vi "AudioTest.Manager.vi"(11 "Module Config":T4={"Name"="Audio Test", "Parent Q"=refnum, "Is Child?"=FALSE, "Index"=0, "Dirs"={"Root"=path "", "Config"=path "C:/ATE/Config", "Logs"=path "C:/ATE/Logs", "Reports"=path "C:/ATE/Reports", "App Data"=path "C:/ProgramData/MAIN"}, "Simulate"=FALSE, "SimCtrl"=refnum}) -> ()   [LabVIEW 2018]
uses:
  <vilib>/KATE/Module/Module Config.ctl
  <vilib>/KATE/Queues/Q.Element.ctl
  <vilib>/KATE/Module/Module.Working Dirs.ctl
  <vilib>/KATE/Event Log/Event Notification/Event Log.Log Level.ctl
  <vilib>/sound2/lvsound2.llb/Sound Data Format.ctl
  <vilib>/KATE/Module/Module.SW Version Info.ctl
  <vilib>/KATE/Module/Window/Window.Task, Action.ctl
  Utils/Functions/FunctMgr/FunctMgr.lvclass
  <vilib>/sound2/lvsound2.llb/Sound Input Task ID.ctl
  <vilib>/sound2/lvsound2.llb/Sampling Mode.ctl
  <vilib>/Utility/sysdir.llb/System Directory Type.ctl
  <vilib>/KATE/Event Log/Event Notification/Event Log.Notification Type.ctl
  <vilib>/sound2/lvsound2.llb/Sound Input Read (DBL).vi
  <vilib>/measure/maspectr.llb/FFT Spectrum (Mag-Phase) for 1 Chan.vi
  <vilib>/KATE/Config/Stored Controls/Class.SaveCtrls.lvclass
  <vilib>/KATE/Queues/Queue Utils.lvlib
  <vilib>/KATE/Module/Module Utils.lvlib
  <vilib>/KATE/Event Log/Event Log.lvlib
  <vilib>/KATE/Scheduler/Scheduler.lvlib
  <vilib>/KATE/Menu/Menu Utils.lvlib
  <vilib>/KATE/Config/Config Utils.lvlib
  <vilib>/KATE/Status/Status Utils.lvlib
  <vilib>/KATE/Files/File Utils.lvlib
  <vilib>/KATE/SeqMgr/SeqMgr.lvlib
  <vilib>/KATE/Event Log/Event Notification/Event Notification.lvclass
  <vilib>/measure/NI_MAPro.lvlib
  <vilib>/KATE/Time/Time Utils.lvlib
panel:
  in  "Main Tab":enum32{"Operate", "Maint"}(tab)
  in  "Data Tab":enum32{"Control", "Config"}(tab)
  out "Dur(s)":dbl=1.0 min=0.1 max=10.0
  out "Recording":bool
  in  "Interval(s)":dbl=1.0 min=0.1 max=10.0
  in  "Read Audio":bool
  in  "Read Baseline":bool
  in  "Save Data to File":bool
  out "Status":string
  in  "Limits":T1(array[cluster])=[{"FreqStart"=0.0, "FreqEnd"=1000.0, "Lim_dB"=-45.0, "Result"=TRUE}, {"FreqStart"=1000.0, "FreqEnd"=8000.0, "Lim_dB"=-60.0, "Result"=TRUE}] {"Lim_dB" format="%#_6f"; "FreqEnd" format="%#.3f"; "FreqStart" format="%#.3f"}
  out "FFT":cluster{"f0":dbl, "df":dbl, "magnitude":dbl[]}[](graph)
  in  "Toggle Sim":bool
  out "Error":errorcluster
  in  "Logging Level":T2
  in  "Audio Format":T3={"sample rate (S/s)"=22050.0, "number of channels"=2, "bits per sample"=16}
  out "Rev":string="v1.0.0"
  out "Simulate Indication":string="Simulating Instruments"
  out "Error Status":string
  in  "Clear Error":bool
  in  "Leave Maint":bool
  # "Audio Test"
  # "Start(Hz)         End(Hz)                    Limit"
  # "P/F"
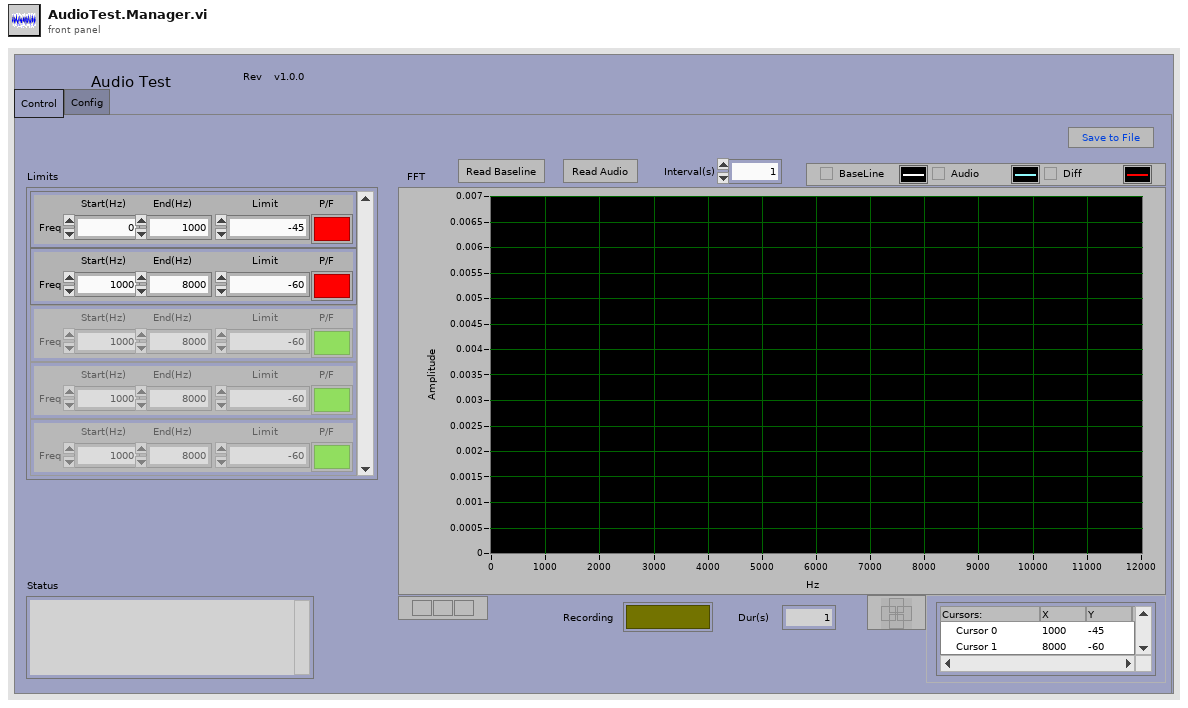
[diagram p1: front panel]
types:
  T1 = cluster{"FreqStart":dbl, "FreqEnd":dbl, "Lim_dB":dbl, "Result":bool}[]
  T2 = typedef "KATE_Lib.lvlib/Event Log.lvlib/Event Log.Log Level.ctl" = enum16{"Normal", "Verbose", "Debug0", "Debug1", "Debug2"}
  T3 = typedef "Sound Data Format.ctl" = cluster{"sample rate (S/s)":dbl, "number of channels":i32, "bits per sample":i32}
  T4 = typedef "KATE_Lib.lvlib/Module Utils.lvlib/Module Config.ctl" = cluster{"Name":string, "Parent Q":refnum<queue>, "Is Child?":bool, "Index":i32, "Dirs":T5, "Simulate":bool, "SimCtrl":refnum<vi>}
  T5 = typedef "KATE_Lib.lvlib/Module Utils.lvlib/Module.Working Dirs.ctl" = cluster{"Root":path, "Config":path, "Logs":path, "Reports":path, "App Data":path}
  T6 = typedef "KATE_Lib.lvlib/Module Utils.lvlib/Module.SW Version Info.ctl" = cluster{"AppName":string, "Company":string, "Version":string, "Description":string, "PN":string}
  T7 = typedef "KATE_Lib.lvlib/Module Utils.lvlib/Module Sys Info.ctl" = cluster{"Main Q":refnum<queue>, "Exe":bool, "SW Rev":T6, "Self Ref":refnum<vi>, "Main Tab":refnum<vi>, "Pane":refnum<vi>, "Stop":cluster{"Ref":refnum<event-registration>, "Event":refnum<user-event>}, "Cfg":T4, "Services":cluster{"Name":string, "vi ref":refnum<vi>}[], "Menu Ref":refnum<k9>, "CtrlStates":refnum<class "Class.SaveCtrls.lvclass">, "Docs":cluster{"Tags":string[], "Paths":path[]}, "Log":refnum<class "Event Notification.lvclass">, "Test Controls":refnum<vi>[], "Child Modules":cluster{"Name":string, "vi ref":refnum<vi>}[], "SW Items":string[][], "AppData":refnum<class "Class.AppData.lvclass">}
  T8 = enum8{"Enabled", "Disabled", "Disabled and Grayed Out"}
  T9 = cluster{"dB On (F)":bool, "unwrap phase (F)":bool, "convert to degree (F)":bool}
  T10 = enum16{"open", "replace", "create", "open or create", "replace or create", "replace or create with confirmation"}
  T11 = cluster{"FreqStart":dbl, "FreqEnd":dbl, "Lim":dbl, "Result":bool}
  T12 = typedef "KATE_Lib.lvlib/Event Log.lvlib/Event Log.Notification Type.ctl" = enum16{"Normal", "Warning", "Error", "Success"}
  T13 = typedef "Sound Input Task ID.ctl" = u32
  T14 = cluster{"Child Modules":cluster{"VI Ref":refnum<vi>, "Name":string}[]}
  T15 = cluster{"Local Error":errorcluster, "Lnch":bool, "FunctMgr":refnum<class "FunctMgr.lvclass">, "App":cluster{"Child Modules":cluster{"VI Ref":refnum<vi>, "Name":string}[]}, "Task ID":T13, "GraphData":cluster{"t":dbl[], "Y":dbl[]}, "Baseline":cluster{"f0":dbl, "df":dbl, "magnitude":dbl[]}, "Audio":cluster{"f0":dbl, "df":dbl, "magnitude":dbl[]}, "Diff":cluster{"f0":dbl, "df":dbl, "magnitude":dbl[]}}
  T16 = typedef "Sampling Mode.ctl" = i32
  T17 = cluster{"FreqStart":dbl, "FreqEnd":dbl, "Lim_dB":dbl, "Result":bool}
  T18 = typedef "System Directory Type.ctl" = i32
  T19 = typedef "KATE_Lib.lvlib/Module Utils.lvlib/Window.Task, Action.ctl" = enum16{"Resize()", "Show Panel(Bool)", "Show Scroll Bars(Bool)", "Dock to SubPanel(SubPanel Ref)", "Undock from SubPanel()", "Return to SubPanel()", "Go To Maint Tab()", "Show Maint Tab(Bool)", "Open Block Diagram()"}
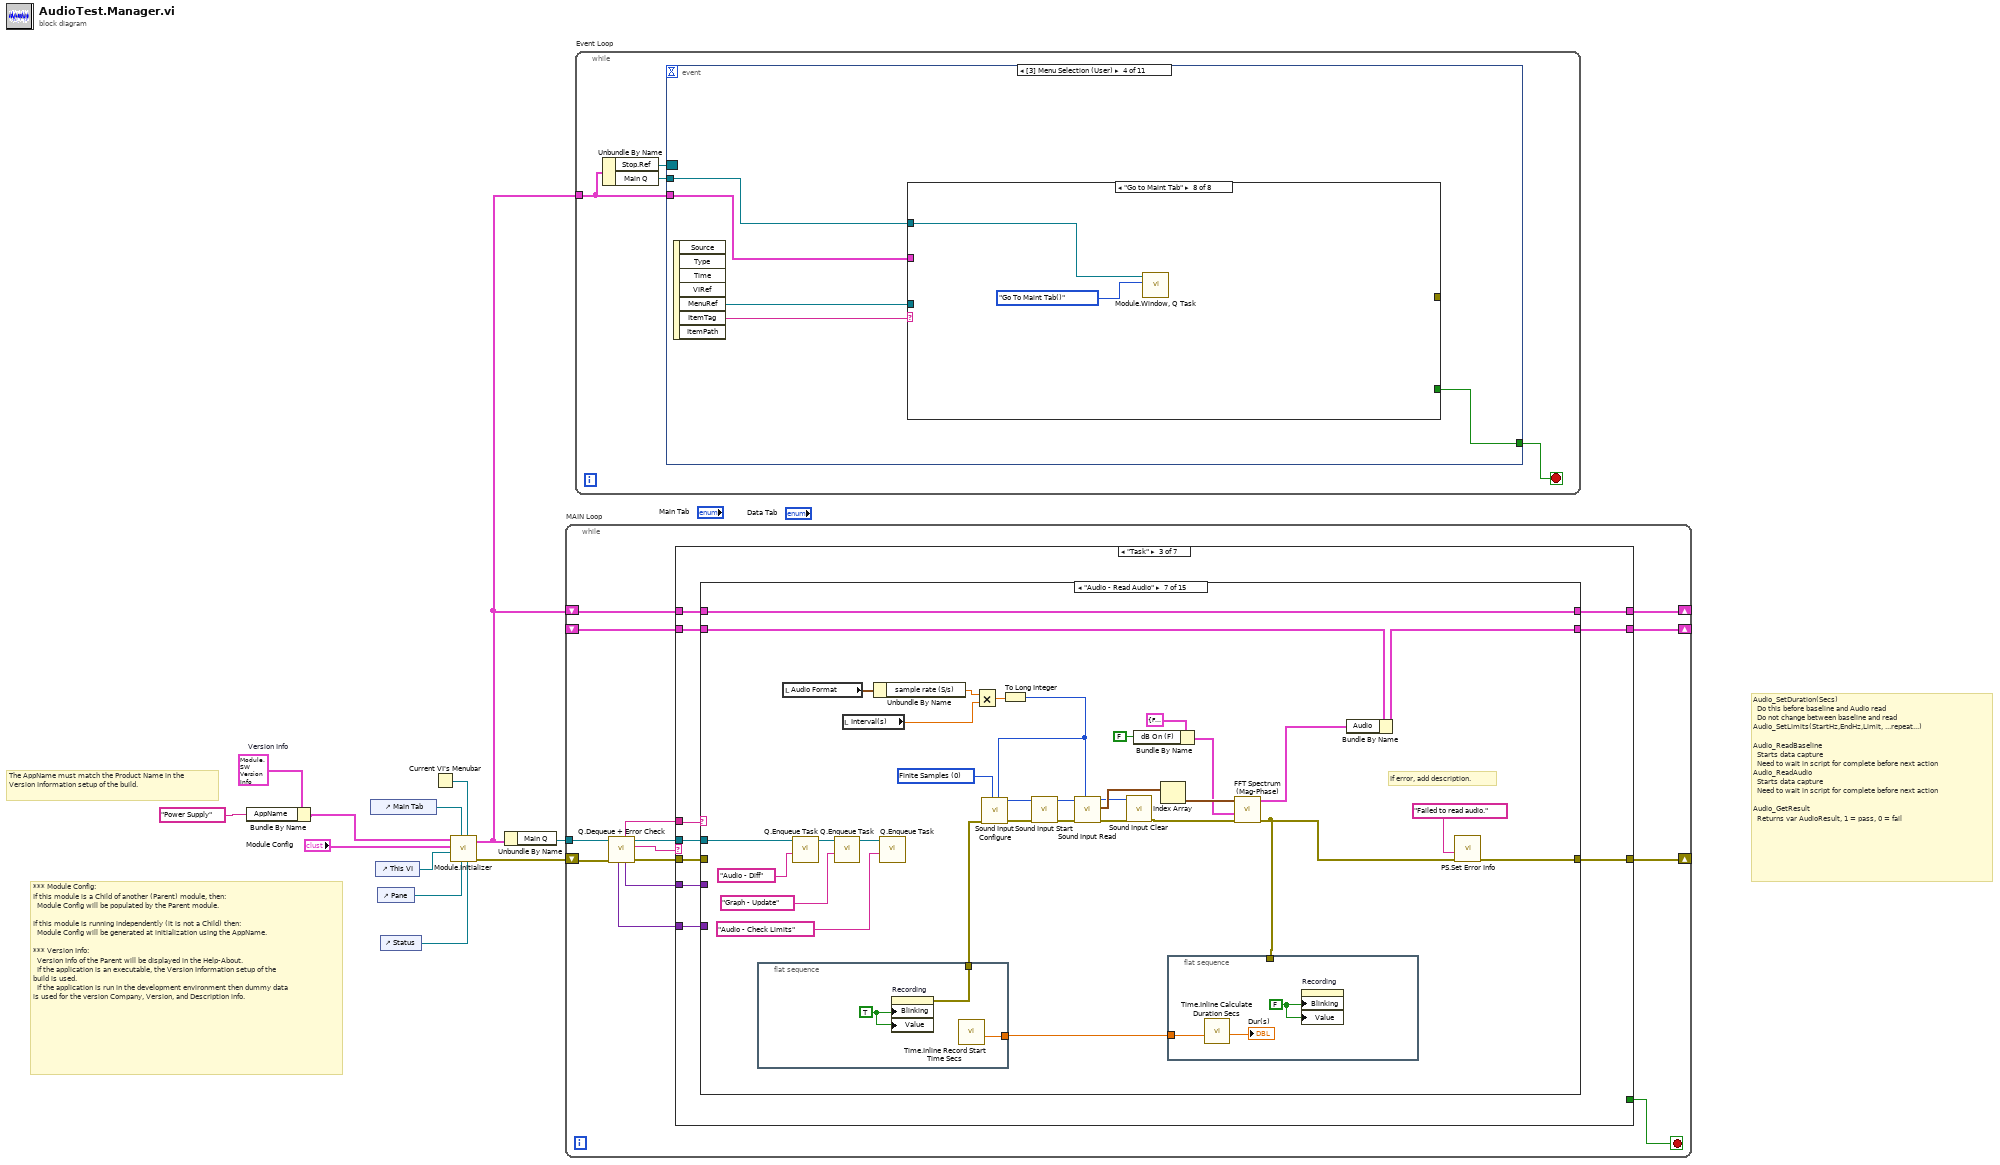
[diagram p0: block diagram]
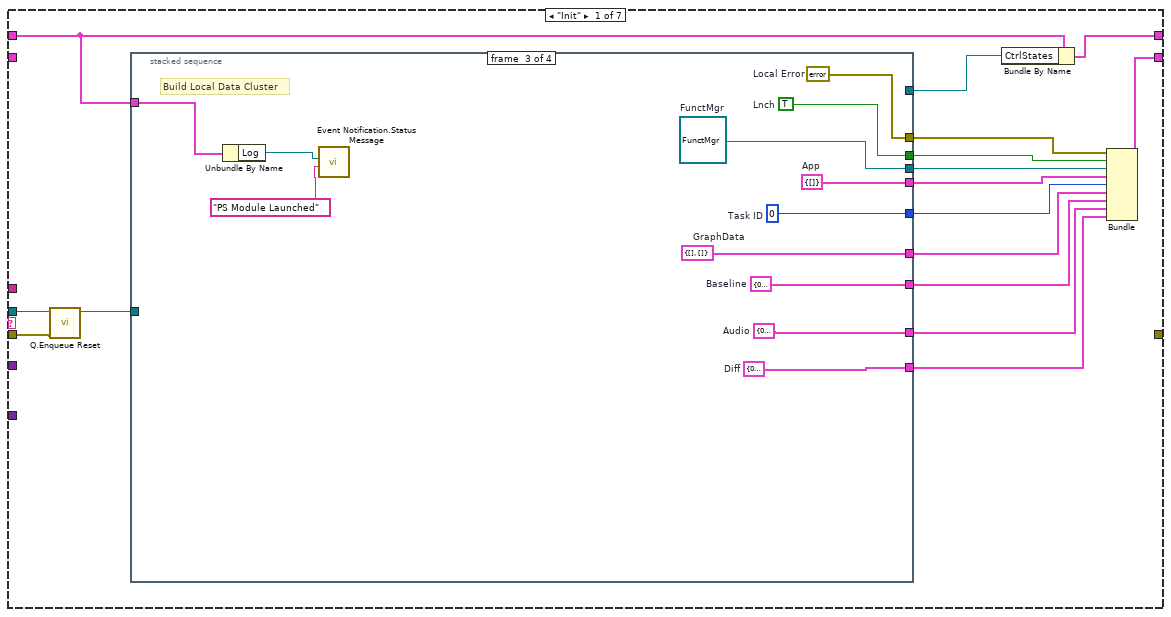
[diagram p2: hidden frame]
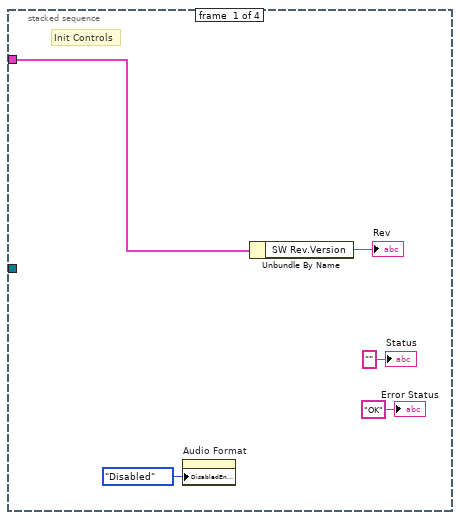
[diagram p3: hidden frame]
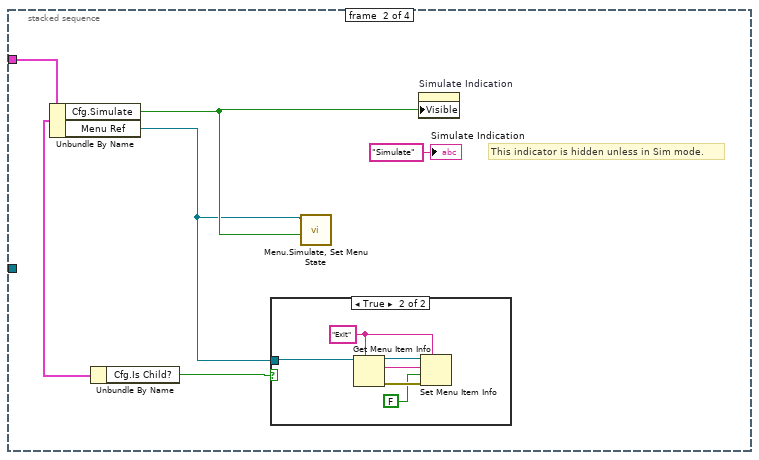
[diagram p4: hidden frame]
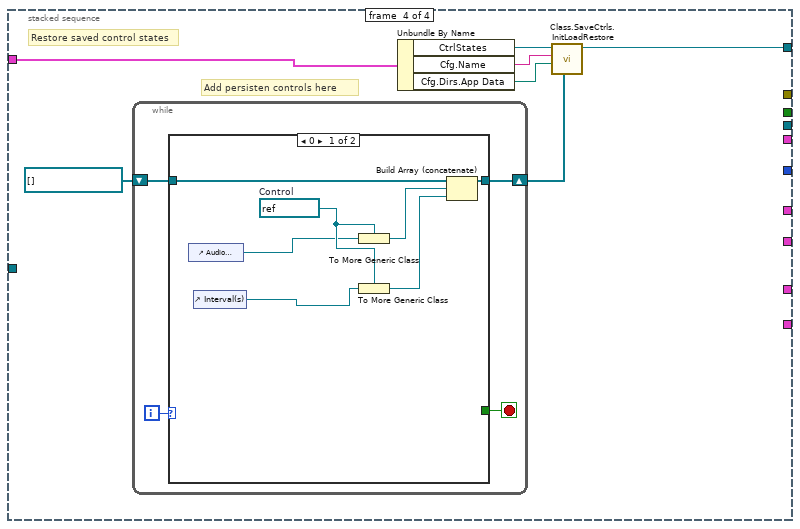
[diagram p6: hidden frame]
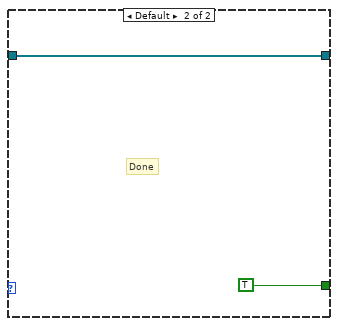
[diagram p7: hidden frame]
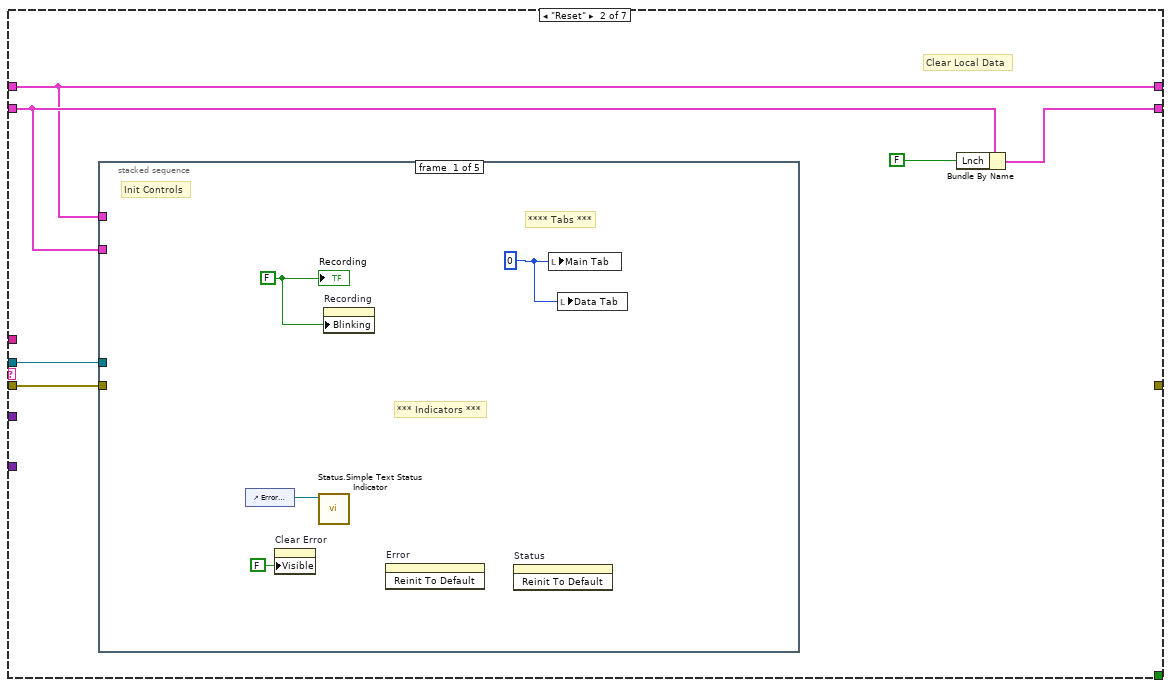
[diagram p8: hidden frame]
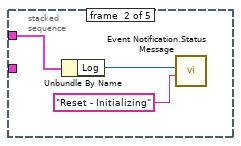
[diagram p9: hidden frame]
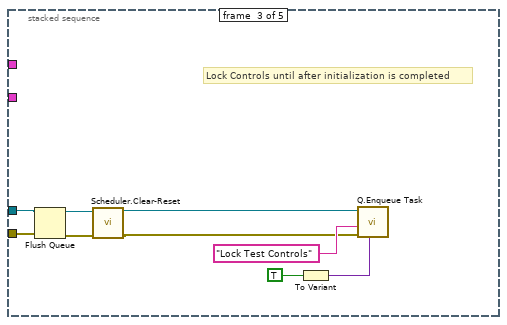
[diagram p10: hidden frame]
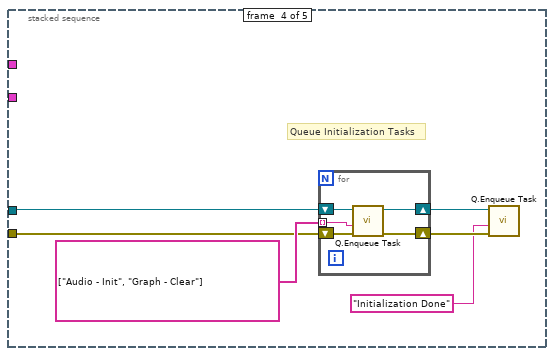
[diagram p11: hidden frame]
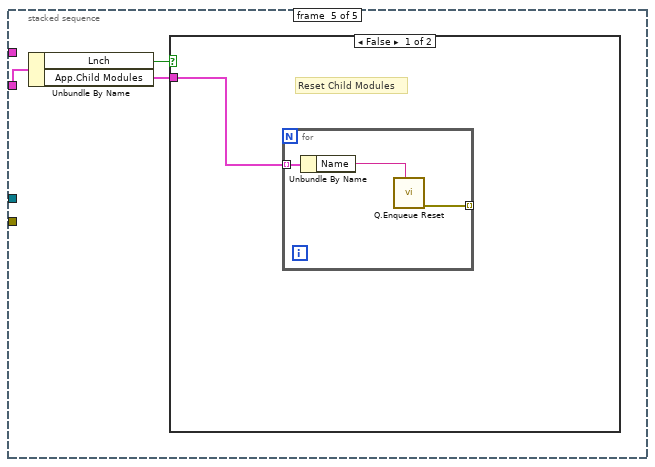
[diagram p12: hidden frame]
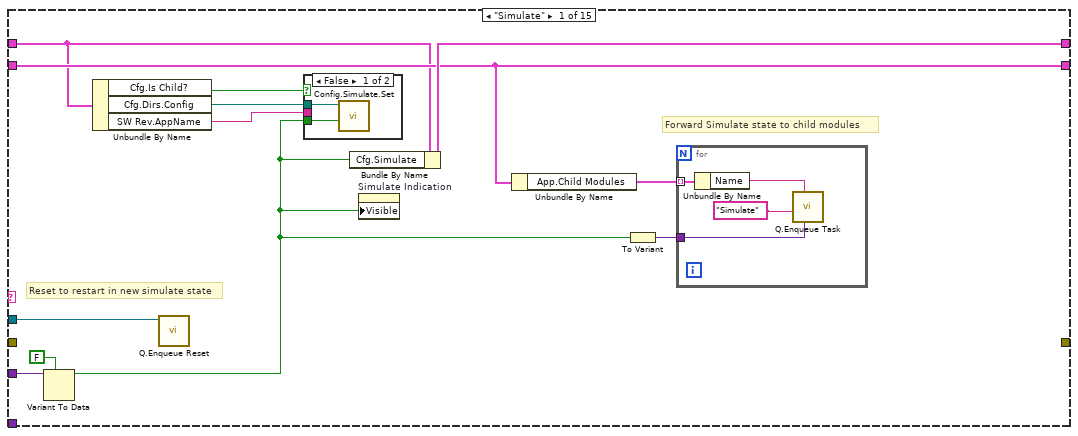
[diagram p14: hidden frame]
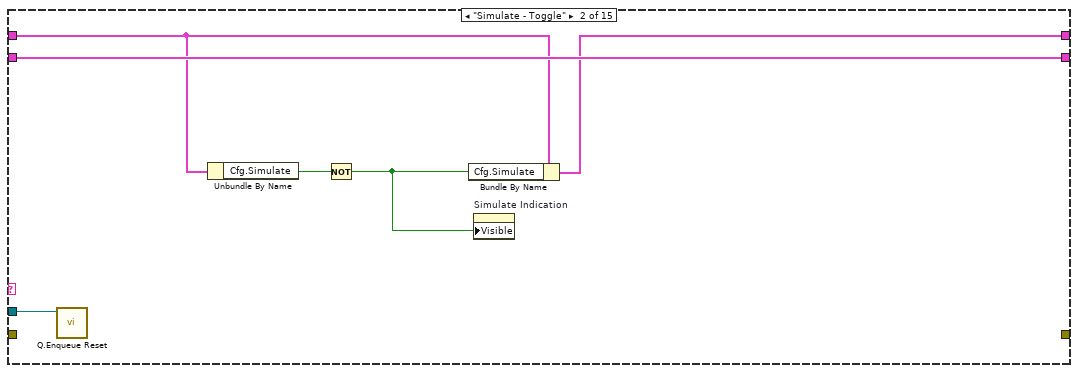
[diagram p16: hidden frame]
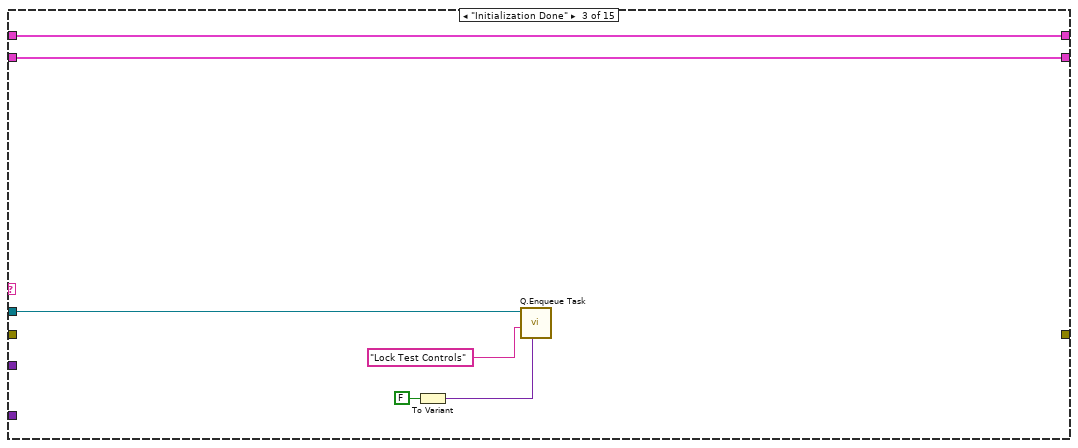
[diagram p17: hidden frame]
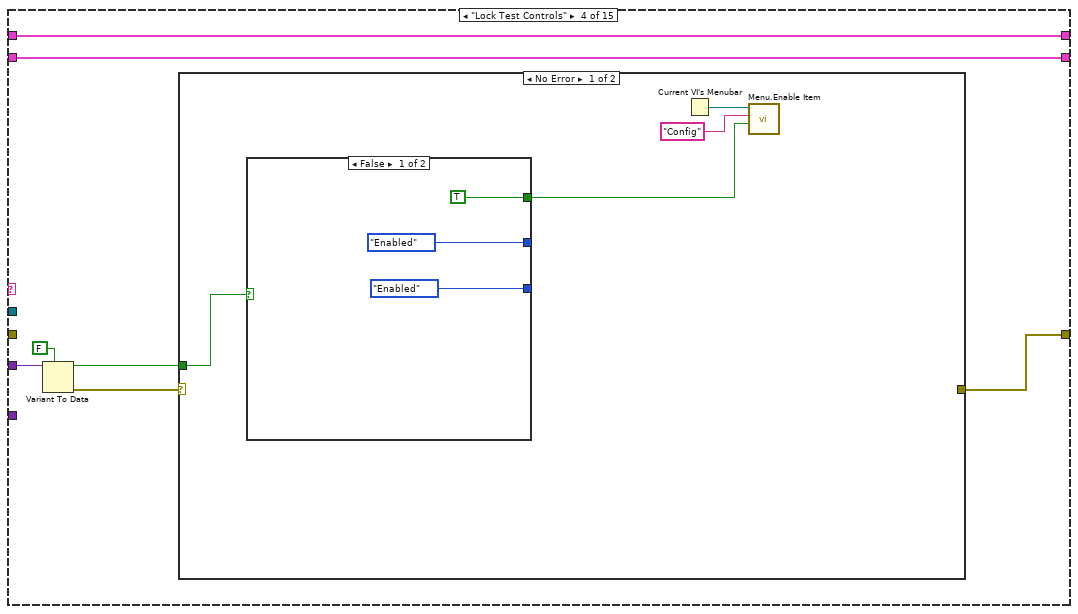
[diagram p18: hidden frame]
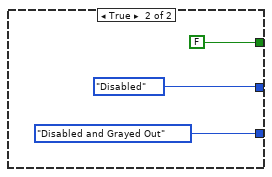
[diagram p19: hidden frame]
diagram:
  w2 = T6 {"AppName"="ModuleX", "Company"="CompanyX", "Version"="1.0", "Description"="This app is being developed.", "PN"=""}  # Version Info
  # "Audio_SetDuration(Secs)\n  Do this before baseline and Audio read\n  Do not change between baseline and read\nAudio_SetLimits(StartHz,EndHz,Limit, ...repeat...)\n\nAudio_ReadBaseline\n  Starts data capture\n  Need to wait in script for complete before next action\nAudio_ReadAudio\n  Starts data capture\n  Need to wait in script for complete before next action\n\nAudio_GetResult\n  Returns var AudioResult, 1 = pass, 0 = fail"
  # "*** Module Config:\nIf this module is a Child of another (Parent) module, then:\n  Module Config will be populated by the Parent module.\n\nIf this module is running independently (it is not a Child) then:\n  Module Config will be generated at initialization using the AppName.\n\n*** Version Info:\n  Version Info of the Parent will be displayed in the Help-About.\n  If the application is an executable, the Version Information setup of the build is used.\n  If the application is run in the development environment then dummy data is used for the version Company, Version, and Description info."
  # "The AppName must match the Product Name in the Version Information setup of the build."
  n1 = Bundle By Name(cluster=w2, "AppName"="Power Supply") -> (w1:T6)
  n2 = control-ref of="Main Tab"() -> (w10:refnum<vi>)
  n3 = control-ref of="This VI"() -> (w9:refnum<vi>)
  n4 = control-ref of="Pane"() -> (w8:refnum<vi>)
  n5 = control-ref of="Status"() -> (w4:refnum<vi>)
  n6 = Current VI's Menubar() -> (w6:refnum<k9>)
  n7 = call <vilib>:"Module.Initializer.vi"("StatusTxtBx"=w4, "Menu Ref"=w6, "Pane"=w8, "Main Tab"=w10, "Self Ref"=w9, "Module Config"="Module Config", "SW Rev"=w1) -> ("error out"=w12:errorcluster, "Sys"=w7:T7)  [unwired: 3 in]
  n8 = Unbundle By Name(w7) -> ("Main Q"=w11:refnum<queue>)
  n9 = while "MAIN Loop" {
    shift-right: [w23] -> _
    shift-left: w12 -> [w21]
    shift-right: [w24] -> _
    shift-left: _ -> [w13]
    shift-right: [w25] -> _
    shift-left: w7 -> [w26]
    tunnel: w11 -> [w20]
    stop <- w15 stop-if-true
    n10 = call <vilib>:"Q.Dequeue + Error Check.vi"("Error In"=w21, "Q In"=w20) -> ("error out"=w22:errorcluster, "Cmd"=w19:string, "Q Out"=w18:refnum<queue>, "Data1"=w17:variant, "Sub"=w14:string, "Data2"=w16:variant)  [unwired: 4 in]
    n11 = case shown="\"Task\"" w19 {
      selector: w19 -> [_ _ _ _ _ w508 _]
      tunnel: w13 -> [_ w93 w139 w407 w482 w502 w567]
      tunnel: w26 -> [w37 w91 w140 w408 w483 w503 w568]
      tunnel: [w38 w91 w138 w406 w481 w503 w568] -> w25
      tunnel: [w40 w96 w137 w405 w480 w501 w567] -> w24
      tunnel: [_ _ w131 w400 _ w509 w570] -> w23
      tunnel: w22 -> [w41 w94 w133 w401 _ w506 _]
      tunnel: w18 -> [w42 w95 w134 w402 w486 w504 _]
      tunnel: w17 -> [_ _ w135 w403 w485 w507 _]
      tunnel: w16 -> [_ _ w132 w399 w484 _ _]
      tunnel: w14 -> [_ _ w136 w404 w487 w505 _]
      tunnel: [_ _ _ _ _ _ TRUE] -> w15
      frame "Init" {
        n12 = call <vilib>:"Q.Enqueue Reset.vi"("Error In"=w41, "Q In"=w42) -> ("Q Out"=w35:refnum<queue>)  [unwired: 8 in, 1 out]
        n13 = stacked-sequence {
          tunnel: [_ _ w64 _] -> w39
          tunnel: w37 -> [w46 w49 w67 w72]
          tunnel: [_ _ _ w71] -> w36
          tunnel: w35 -> [_ _ _ _]
          tunnel: [_ _ w70 _] -> w34
          tunnel: [_ _ w69 _] -> w33
          tunnel: [_ _ w62 _] -> w32
          tunnel: [_ _ w68 _] -> w31
          tunnel: [_ _ w63 _] -> w30
          tunnel: [_ _ w61 _] -> w29
          tunnel: [_ _ w60 _] -> w28
          tunnel: [_ _ w59 _] -> w27
          frame #0 {
            # "Init Controls"
            n14 = property on="Audio Format" class="Clust (strict)"("DisabledEnum"=T8."Disabled" ("Disabled")) -> ()  [unwired: 2 in, 2 out]
            n15 = Unbundle By Name(w46) -> ("SW Rev.Version"=→"Rev":string)
            "Status" <- "" ("Status")
            "Error Status" <- "OK" ("Error Status")
          }
          frame #1 {
            # "This indicator is hidden unless in Sim mode."
            n16 = Unbundle By Name(w49) -> ("Cfg.Simulate"=w51:bool, "Menu Ref"=w48:refnum<k9>)
            n17 = Unbundle By Name(w49) -> ("Cfg.Is Child?"=w50:bool)
            n18 = case shown="True" w50 {
              tunnel: w48 -> [_ w54]
              frame False {
              }
              frame True {
                w56 = "Exit"
                n19 = Get Menu Item Info(7:w56, 11:w54) -> (0:w55:errorcluster, 2:w57:string, 3:w58:refnum<k9>)  [unwired: 1 in, 4 out]
                n20 = Set Menu Item Info(7:w56, 8:w55, 9:FALSE ("enabled"), 10:w57, 11:w58) -> ()  [unwired: 2 in, 2 out]
              }
            }
            n21 = call <vilib>:"Menu.Simulate, Set Menu State.vi"("Sim Enable"=w51, "Menu Ref"=w48) -> ()  [unwired: 8 in, 2 out]
            n22 = property on="Simulate Indication" class="Str"("Visible"=w51) -> ()  [unwired: 2 in, 2 out]
            "Simulate Indication" <- "Simulate" ("Simulate Indication")
          }
          frame #2 {
            w59 = cluster{"f0":dbl, "df":dbl, "magnitude":dbl[]} {"f0"=0.0, "df"=0.0, "magnitude"=[]}  # Diff
            w60 = cluster{"f0":dbl, "df":dbl, "magnitude":dbl[]} {"f0"=0.0, "df"=0.0, "magnitude"=[]}  # Audio
            w61 = cluster{"f0":dbl, "df":dbl, "magnitude":dbl[]} {"f0"=0.0, "df"=0.0, "magnitude"=[]}  # Baseline
            w62 = T13 0  # Task ID
            w63 = cluster{"t":dbl[], "Y":dbl[]} {"t"=[], "Y"=[]}  # GraphData
            w68 = errorcluster {"status"=FALSE, "code"=0, "source"=""}  # Local Error
            w64 = refnum<class "FunctMgr.lvclass"> refnum  # FunctMgr
            w69 = T14 {"Child Modules"=[]}  # App
            w70 = TRUE  # Lnch
            # "Build Local Data Cluster"
            n23 = Unbundle By Name(w67) -> ("Log"=w66:refnum<class "Event Notification.lvclass">)
            n24 = call <vilib>:"Event Notification.Status Message.vi"("Message"="PS Module Launched", "Event Notification in"=w66) -> ()  [unwired: 10 in]
          }
          frame #3 {
            # "Add persisten controls here"
            # "Restore saved control states"
            n25 = while {
              shift-right: [w79] -> w73
              shift-left: refnum<vi>[] [] -> [w80]
              i -> [w81]
              stop <- w78 stop-if-true
              n26 = case shown="0" w81 {
                tunnel: w80 -> [w87 w90]
                tunnel: [w88 w90] -> w79
                tunnel: [_ TRUE] -> w78
                frame 0 {
                  w84 = refnum<vi> refnum  # Control
                  n27 = control-ref of="Audio Format"() -> (w83:refnum<vi>)
                  n28 = control-ref of="Interval(s)"() -> (w82:refnum<vi>)
                  n29 = To More Generic Class(target class=w84, reference=w83) -> (generic class reference=w86:refnum<vi>)
                  n30 = To More Generic Class(target class=w84, reference=w82) -> (generic class reference=w85:refnum<vi>)
                  n31 = Build Array (concatenate)(w87, w86, w85) -> (w88:refnum<vi>[])
                }
                frame Default {
                  # "Done"
                }
              }
            }
            n32 = Unbundle By Name(w72) -> ("CtrlStates"=w74:refnum<class "Class.SaveCtrls.lvclass">, "Cfg.Name"=w76:string, "Cfg.Dirs.App Data"=w75:path)
            n33 = call-dynamic "Class.SaveCtrls.InitLoadRestore.vi"("Ctrl Array"=w73, "Module Data Dir"=w75, "Module Name"=w76, "CtrlStates In"=w74) -> ("CtrlStates"=w71:refnum<class "Class.SaveCtrls.lvclass">)  [unwired: 6 in, 1 out]
          }
        }
        n34 = Bundle By Name(cluster=w37, "CtrlStates"=w36) -> (w38:T7)
        n35 = Bundle("Local Error"=w31, "Lnch"=w34, "FunctMgr"=w39, "App"=w33, "Task ID"=w32, "GraphData"=w30, "Baseline"=w29, "Audio"=w28, "Diff"=w27) -> (w40:T15)  [unwired: 1 in]
      }
      frame "Reset" {
        # "Clear Local Data"
        n36 = stacked-sequence {
          tunnel: w95 -> [_ _ w105 w113 _]
          tunnel: w94 -> [_ _ w104 w117 _]
          tunnel: w93 -> [_ _ _ _ w126]
          tunnel: w91 -> [_ w103 _ _ _]
          frame #0 {
            w97 = FALSE ("Recording")
            w100 = 0
            # "*** Indicators ***"
            # "**** Tabs ***"
            # "Init Controls"
            n37 = control-ref of="Error Status"() -> (w99:refnum<vi>)
            n38 = property on="Clear Error" class="Bool"("Visible"=FALSE) -> ()  [unwired: 2 in, 2 out]
            n39 = call <vilib>:"Status.Simple Text Status Indicator.vi"("Status TextBox"=w99) -> ()  [unwired: 10 in, 1 out]
            n40 = property on="Recording" class="Bool (strict)"("Blinking"=w97) -> ()  [unwired: 2 in, 2 out]
            n41 = invoke on="Error" class="Clust (strict)" method="Reinit To Default"() -> ()  [unwired: 3 in, 3 out]
            n42 = invoke on="Status" class="Str" method="Reinit To Default"() -> ()  [unwired: 3 in, 3 out]
            n43 = local write "Main Tab"(w100) -> ()
            n44 = local write "Data Tab"(w100) -> ()
            "Recording" <- w97
          }
          frame #1 {
            n45 = Unbundle By Name(w103) -> ("Log"=w102:refnum<class "Event Notification.lvclass">)
            n46 = call <vilib>:"Event Notification.Status Message.vi"("Message"="Reset - Initializing", "Event Notification in"=w102) -> ()  [unwired: 10 in]
          }
          frame #2 {
            # "Lock Controls until after initialization is completed"
            n47 = Flush Queue(queue=w105, error in (no error)=w104) -> (queue out=w106:refnum<queue>, error out=w109:errorcluster)  [unwired: 1 out]
            n48 = call <vilib>:"Scheduler.Clear-Reset.vi"("error in"=w109, "Q In"=w106) -> ("error out"=w107:errorcluster, "Q Out"=w108:refnum<queue>)  [unwired: 8 in]
            n49 = To Variant(anything=TRUE) -> (Variant=w111:variant)
            n50 = call <vilib>:"Q.Enqueue Task.vi"("Data1"=w111, "Error In"=w107, "Task Name"="Lock Test Controls", "Q In"=w108) -> ()  [unwired: 6 in, 2 out]
          }
          frame #3 {
            # "Queue Initialization Tasks"
            n51 = for {
              shift-right: [w121] -> w115
              shift-left: w117 -> [w122]
              tunnel: string[] ["Audio - Init", "Graph - Clear"] -> [w119] mode=indexing
              shift-right: [w120] -> w116
              shift-left: w113 -> [w123]
              n52 = call <vilib>:"Q.Enqueue Task.vi"("Error In"=w122, "Task Name"=w119, "Q In"=w123) -> ("error out"=w121:errorcluster, "Q Out"=w120:refnum<queue>)  [unwired: 7 in]
            }
            n53 = call <vilib>:"Q.Enqueue Task.vi"("Error In"=w115, "Task Name"="Initialization Done", "Q In"=w116) -> ()  [unwired: 7 in, 2 out]
          }
          frame #4 {
            n54 = Unbundle By Name(w126) -> ("Lnch"=w125:bool, "App.Child Modules"=w124:cluster{"VI Ref":refnum<vi>, "Name":string}[])
            n55 = case shown="False" w125 {
              tunnel: w124 -> [w127 _]
              frame False {
                # "Reset Child Modules"
                n56 = for {
                  tunnel: w127 -> [w130] mode=indexing
                  tunnel: [w128] -> _ mode=indexing
                  n57 = Unbundle By Name(w130) -> ("Name"=w129:string)
                  n58 = call <vilib>:"Q.Enqueue Reset.vi"("Q Name"=w129) -> ("error out"=w128:errorcluster)  [unwired: 9 in, 1 out]
                }
              }
              frame True {
                # "Do not reset at launch.\nThey are already reset"
              }
            }
          }
        }
        n59 = Bundle By Name(cluster=w93, "Lnch"=FALSE ("Test.Running")) -> (w96:T15)
      }
      frame "Task" {
        n60 = case shown="\"Audio - Read Audio\"" w136 {
          selector: w136 -> [_ _ _ _ _ _ _ _ _ _ _ _ _ _ w393]
          tunnel: w140 -> [w145 w161 w170 w177 w190 w220 w259 w276 w286 w319 w321 w355 w366 w379 w394]
          tunnel: w139 -> [w149 w163 w165 w171 w189 w210 w246 w272 w278 w318 w320 w354 w362 w378 w395]
          tunnel: [w150 w162 w170 w177 w190 w220 w259 w276 w286 w319 w321 w355 w366 w379 w394] -> w138
          tunnel: [w149 w163 w165 w171 w189 w209 w250 w271 w278 w318 w320 w354 w361 w378 w395] -> w137
          tunnel: w135 -> [w152 _ _ w176 _ _ _ _ _ _ _ _ w358 w380 w392]
          tunnel: w134 -> [w146 w164 w169 _ _ w206 w248 _ _ _ _ _ _ _ _]
          tunnel: w133 -> [_ _ _ _ _ _ _ _ _ _ _ _ _ _ w390]
          tunnel: w132 -> [_ _ _ _ _ _ _ _ _ _ _ _ w359 _ w391]
          tunnel: [_ _ _ w173 w192 w221 w260 _ _ _ _ _ w360 w377 w389] -> w131
          frame "Simulate" {
            # "Reset to restart in new simulate state"
            # "Forward Simulate state to child modules"
            n61 = Variant To Data(type=FALSE, Variant=w152) -> (data=w142:bool)  [unwired: 1 in, 1 out]
            n62 = Unbundle By Name(w145) -> ("Cfg.Is Child?"=w141:bool, "Cfg.Dirs.Config"=w144:path, "SW Rev.AppName"=w143:string)
            n63 = call <vilib>:"Q.Enqueue Reset.vi"("Q In"=w146) -> ()  [unwired: 9 in, 2 out]
            n64 = case shown="False" w141 {
              tunnel: w144 -> [w154 _]
              tunnel: w143 -> [_ _]
              tunnel: w142 -> [w153 _]
              frame False {
                n65 = call <vilib>:"Config.Simulate.Set.vi"("Simulate"=w153, "Config Folder"=w154) -> ()  [unwired: 9 in, 1 out]
              }
              frame True {
              }
            }
            n66 = Bundle By Name(cluster=w145, "Cfg.Simulate"=w142) -> (w150:T7)
            n67 = property on="Simulate Indication" class="Str"("Visible"=w142) -> ()  [unwired: 2 in, 2 out]
            n68 = Unbundle By Name(w149) -> ("App.Child Modules"=w148:cluster{"VI Ref":refnum<vi>, "Name":string}[])
            n69 = To Variant(anything=w142) -> (Variant=w147:variant)
            n70 = for {
              tunnel: w148 -> [w158] mode=indexing
              tunnel: w147 -> [w155]
              n71 = Unbundle By Name(w158) -> ("Name"=w157:string)
              n72 = call <vilib>:"Q.Enqueue Task.vi"("Data1"=w155, "Q Name"=w157, "Task Name"="Simulate") -> ()  [unwired: 7 in, 2 out]
            }
          }
          frame "Simulate - Toggle" {
            n73 = call <vilib>:"Q.Enqueue Reset.vi"("Q In"=w164) -> ()  [unwired: 9 in, 2 out]
            n74 = Unbundle By Name(w161) -> ("Cfg.Simulate"=w160:bool)
            n75 = Not(x=w160) -> (.not. x?=w159:bool)
            n76 = Bundle By Name(cluster=w161, "Cfg.Simulate"=w159) -> (w162:T7)
            n77 = property on="Simulate Indication" class="Str"("Visible"=w159) -> ()  [unwired: 2 in, 2 out]
          }
          frame "Initialization Done" {
            n78 = To Variant(anything=FALSE) -> (Variant=w167:variant)
            n79 = call <vilib>:"Q.Enqueue Task.vi"("Data1"=w167, "Task Name"="Lock Test Controls", "Q In"=w169) -> ()  [unwired: 7 in, 2 out]
          }
          frame "Lock Test Controls" {
            n80 = Variant To Data(type=FALSE, Variant=w176) -> (data=w172:bool, error out=w174:errorcluster)  [unwired: 1 in]
            n81 = case shown="No Error" w174 {
              selector: w174 -> [_ w188]
              tunnel: w172 -> [w181 _]
              tunnel: [_ w188] -> w173
              frame No Error {
                n82 = case shown="False" w181 {
                  tunnel: [T8."Enabled" ("Disabled") T8."Disabled and Grayed Out" ("Disabled")] -> _
                  tunnel: [T8."Enabled" ("Disabled") T8."Disabled" ("Disabled")] -> _
                  tunnel: [TRUE ("Enable") FALSE ("Enable")] -> w178
                  frame False {
                  }
                  frame True {
                  }
                }
                n83 = Current VI's Menubar() -> (w179:refnum<k9>)
                n84 = call <vilib>:"Menu.Enable Item.vi"("Enable"=w178, "Tag"="Config", "Menu Ref"=w179) -> ()  [unwired: 7 in, 2 out]
              }
              frame Error {
              }
            }
          }
          frame "Audio - Init" {
            n85 = call "PS.Set Error Info.vi"("Description"="Failed to init default audio input device.") -> ("error out"=w192:errorcluster)  [unwired: 10 in]
          }
          frame "Audio - Read Baseline" {
            w199 = T16 0 items=["Finite Samples", "Continuous Samples"] ("sample mode")
            # "If error, add description."
            n86 = local read "Audio Format"() -> (w212:T3)
            n87 = flat-sequence {
              tunnel: [w227] -> w194
              tunnel: [w226] -> w193
              frame #0 {
                w228 = TRUE
                n88 = property on="Recording" class="Bool (strict)"("Blinking"=w228, "Value"=w228) -> (error out=w227:errorcluster)  [unwired: 2 in, 1 out]
                n89 = call <vilib>:"Time.Inline Record Start Time Secs.vi"() -> ("Start(s)"=w226:dbl)  [unwired: 9 in, 2 out]
              }
            }
            n90 = Unbundle By Name(w212) -> ("sample rate (S/s)"=w213:dbl)
            n91 = call <vilib>:"Q.Enqueue Task.vi"("Task Name"="Graph - Update" ("Name"), "Q In"=w206) -> ()  [unwired: 8 in, 2 out]
            n92 = Multiply(x=w213, y="Interval(s)") -> (x*y=w215:dbl)
            n93 = To Long Integer(number=w215) -> (32bit integer=w200:i32)
            n94 = call <vilib>:"Sound Input Configure.vi"("number of samples/ch"=w200, "sample mode"=w199, "error in (no error)"=w194) -> ("error out"=w201:errorcluster, "task ID"=w202:T13)  [unwired: 7 in]
            n95 = call <vilib>:"Sound Input Start.vi"("error in (no error)"=w201, "task ID"=w202) -> ("error out"=w203:errorcluster, "task ID out"=w204:T13)  [unwired: 8 in]
            n96 = call-poly <vilib>:"Sound Input Read.vi"("number of samples/ch"=w200, "error in (no error)"=w203, "task ID"=w204) -> ("error out"=w198:errorcluster, "data"=w205:waveform(dbl)[], "task ID out"=w197:T13)  [unwired: 6 in]
            n97 = Bundle By Name(cluster=T9 {"dB On (F)"=FALSE, "unwrap phase (F)"=FALSE, "convert to degree (F)"=FALSE} ("view"), "dB On (F)"=FALSE) -> (w217:T9)
            n98 = call <vilib>:"Sound Input Clear.vi"("error in (no error)"=w198, "task ID"=w197) -> ("error out"=w196:errorcluster)  [unwired: 9 in]
            n99 = Index Array(array=w205) -> (element=w219:waveform(dbl))  [unwired: 1 in]
            n100 = call-poly <vilib>:"FFT Spectrum (Mag-Phase).vi"("error in (no error)"=w196, "view"=w217, "time signal"=w219) -> ("error out"=w195:errorcluster, "magnitude"=w211:cluster{"f0":dbl, "df":dbl, "magnitude":dbl[]})  [unwired: 4 in, 3 out]
            n101 = Bundle By Name(cluster=w210, "Audio"=cluster{"f0":dbl, "df":dbl, "magnitude":dbl[]} {"f0"=0.0, "df"=0.0, "magnitude"=[]}, "Baseline"=w211) -> (w209:T15)
            n102 = flat-sequence {
              tunnel: w195 -> [_]
              tunnel: w193 -> [w224]
              frame #0 {
                w225 = FALSE ("Recording")
                n103 = call <vilib>:"Time.Inline Calculate Duration Secs.vi"("Start(Sec)"=w224) -> ("Duration(s)"=w223:dbl)  [unwired: 8 in, 2 out]
                n104 = local write "Dur(s)"(w223) -> ()
                n105 = property on="Recording" class="Bool (strict)"("Blinking"=w225, "Value"=w225) -> ()  [unwired: 2 in, 2 out]
              }
            }
            n106 = call "PS.Set Error Info.vi"("error in"=w195, "Description"="Failed to read audio.") -> ("error out"=w221:errorcluster)  [unwired: 9 in]
          }
          frame "Audio - Read Audio" {
            w237 = T16 0 items=["Finite Samples", "Continuous Samples"] ("sample mode")
            # "If error, add description."
            n107 = flat-sequence {
              tunnel: [w266] -> w231
              tunnel: [w265] -> w229
              frame #0 {
                w267 = TRUE ("Recording")
                n108 = property on="Recording" class="Bool (strict)"("Blinking"=w267, "Value"=w267) -> (error out=w266:errorcluster)  [unwired: 2 in, 1 out]
                n109 = call <vilib>:"Time.Inline Record Start Time Secs.vi"() -> ("Start(s)"=w265:dbl)  [unwired: 9 in, 2 out]
              }
            }
            n110 = local read "Audio Format"() -> (w252:T3)
            n111 = call <vilib>:"Q.Enqueue Task.vi"("Task Name"="Audio - Diff" ("Name"), "Q In"=w248) -> ("Q Out"=w245:refnum<queue>)  [unwired: 8 in, 1 out]
            n112 = call <vilib>:"Q.Enqueue Task.vi"("Task Name"="Graph - Update" ("Name"), "Q In"=w245) -> ("Q Out"=w243:refnum<queue>)  [unwired: 8 in, 1 out]
            n113 = local read "Interval(s)"() -> (w247:dbl)
            n114 = Unbundle By Name(w252) -> ("sample rate (S/s)"=w253:dbl)
            n115 = call <vilib>:"Q.Enqueue Task.vi"("Task Name"="Audio - Check Limits" ("Name"), "Q In"=w243) -> ()  [unwired: 8 in, 2 out]
            n116 = Multiply(x=w253, y=w247) -> (x*y=w254:dbl)
            n117 = To Long Integer(number=w254) -> (32bit integer=w235:i32)
            n118 = call <vilib>:"Sound Input Configure.vi"("number of samples/ch"=w235, "sample mode"=w237, "error in (no error)"=w231) -> ("error out"=w238:errorcluster, "task ID"=w239:T13)  [unwired: 7 in]
            n119 = call <vilib>:"Sound Input Start.vi"("error in (no error)"=w238, "task ID"=w239) -> ("error out"=w240:errorcluster, "task ID out"=w241:T13)  [unwired: 8 in]
            n120 = call-poly <vilib>:"Sound Input Read.vi"("number of samples/ch"=w235, "error in (no error)"=w240, "task ID"=w241) -> ("error out"=w234:errorcluster, "data"=w236:waveform(dbl)[], "task ID out"=w232:T13)  [unwired: 6 in]
            n121 = call <vilib>:"Sound Input Clear.vi"("error in (no error)"=w234, "task ID"=w232) -> ("error out"=w233:errorcluster)  [unwired: 9 in]
            n122 = Bundle By Name(cluster=T9 {"dB On (F)"=FALSE, "unwrap phase (F)"=FALSE, "convert to degree (F)"=FALSE} ("view"), "dB On (F)"=FALSE) -> (w256:T9)
            n123 = Index Array(array=w236) -> (element=w258:waveform(dbl))  [unwired: 1 in]
            n124 = flat-sequence {
              tunnel: w230 -> [_]
              tunnel: w229 -> [w263]
              frame #0 {
                w264 = FALSE ("Recording")
                n125 = call <vilib>:"Time.Inline Calculate Duration Secs.vi"("Start(Sec)"=w263) -> ("Duration(s)"=→"Dur(s)":dbl)  [unwired: 8 in, 2 out]
                n126 = property on="Recording" class="Bool (strict)"("Blinking"=w264, "Value"=w264) -> ()  [unwired: 2 in, 2 out]
              }
            }
            n127 = call-poly <vilib>:"FFT Spectrum (Mag-Phase).vi"("error in (no error)"=w233, "view"=w256, "time signal"=w258) -> ("error out"=w230:errorcluster, "magnitude"=w251:cluster{"f0":dbl, "df":dbl, "magnitude":dbl[]})  [unwired: 4 in, 3 out]
            n128 = Bundle By Name(cluster=w246, "Audio"=w251) -> (w250:T15)
            n129 = call "PS.Set Error Info.vi"("error in"=w230, "Description"="Failed to read audio.") -> ("error out"=w260:errorcluster)  [unwired: 9 in]
          }
          frame "Audio - Diff" {
            n130 = Unbundle By Name(w272) -> ("Audio"=w273:cluster{"f0":dbl, "df":dbl, "magnitude":dbl[]}, "Audio.magnitude"=w275:dbl[], "Baseline.magnitude"=w274:dbl[])
            n131 = Subtract(x=w275, y=w274) -> (x-y=w268:dbl[])
            n132 = Absolute Value(x=w268) -> (abs(x)=w269:dbl[])
            n133 = Bundle By Name(cluster=w273, "magnitude"=w269) -> (w270:cluster{"f0":dbl, "df":dbl, "magnitude":dbl[]})
            n134 = Bundle By Name(cluster=w272, "Diff"=w270) -> (w271:T15)
          }
          frame "Audio - Check Limits" {
            n135 = Unbundle By Name(w278) -> ("Diff"=w277:cluster{"f0":dbl, "df":dbl, "magnitude":dbl[]})
            n136 = Unbundle By Name(w277) -> ("magnitude"=w285:dbl[], "f0"=w284:dbl, "df"=w283:dbl)
            n137 = for {
              tunnel: w285 -> [w289] mode=indexing
              tunnel: w284 -> [w291]
              tunnel: w283 -> [w293]
              tunnel: [w290] -> w281 mode=indexing
              tunnel: [w289] -> w282 mode=indexing
              i -> [w288]
              n138 = To Double Precision Float(number=w288) -> (double precision float=w287:dbl)
              n139 = Multiply(x=w293, y=w287) -> (x*y=w292:dbl)
              n140 = Add(x=w291, y=w292) -> (x+y=w290:dbl)
            }
            n141 = for {
              tunnel: "Limits" -> [w306] mode=indexing
              tunnel: w282 -> [w311]
              tunnel: w281 -> [w313]
              tunnel: [w308] -> w280 mode=indexing
              tunnel: [w296] -> _
              i -> [w294]
              n142 = Unbundle By Name(w306) -> ("Lim_dB"=w297:dbl, "FreqEnd"=w305:dbl, "FreqStart"=w304:dbl)
              n143 = Max & Min(x=w305, y=w304) -> (max(x,y)=w298:dbl, min(x,y)=w303:dbl)
              n144 = Threshold 1D Array(2:w298, 3:w313) -> (0:w312:dbl)  [unwired: 1 in]
              n145 = Threshold 1D Array(2:w303, 3:w313) -> (0:w299:dbl)  [unwired: 1 in]
              n146 = Subtract(x=w312, y=w299) -> (x-y=w302:dbl)
              n147 = To Long Integer(number=w299) -> (32bit integer=w300:i32)
              n148 = To Long Integer(number=w302) -> (32bit integer=w301:i32)
              n149 = Array Subset(array=w311, index=w300, length=w301) -> (w310:dbl[])
              n150 = To Unsigned Long Integer(number=w294) -> (unsigned 32bit integer=w295:u32)
              n151 = Array Max & Min(array=w310) -> (max value=w309:dbl)  [unwired: 3 out]
              n152 = Greater?(x=w309, y=w297) -> (0:w307:bool)
              n153 = Bundle By Name(cluster=w306, "Result"=w307) -> (w308:T17)
              n154 = property on="FFT" class="WFGraph (strict)"("Active Cursor"=w295, "Cursor.Cursor X"=w298, "Cursor.Cursor Y"=w297) -> (error out=w296:errorcluster)  [unwired: 2 in, 1 out]
            }
            n155 = local write "Limits"(w280) -> ()
          }
          frame "Graph - Update" {
            n156 = Unbundle By Name(w318) -> ("Baseline"=w317:cluster{"f0":dbl, "df":dbl, "magnitude":dbl[]}, "Audio"=w316:cluster{"f0":dbl, "df":dbl, "magnitude":dbl[]}, "Diff"=w315:cluster{"f0":dbl, "df":dbl, "magnitude":dbl[]})
            n157 = Build Array(w317, w316, w315) -> (→"FFT":cluster{"f0":dbl, "df":dbl, "magnitude":dbl[]}[])
          }
          frame "Graph - Clear" {
          }
          frame "Save Data to File" {
            w344 = T18 2 items=["User Home"=0, "User Desktop"=1, "User Documents"=2, "User Application Data"=3, "User Preferences"=4, "User Temporary"=5, "Public Documents"=6, "Public Application Data"=7, "Public Preferences"=8, "Public Cache"=13, "System Core Libraries"=9, "System Installed Libraries"=10, "Application Files"=11, "Boot Volume Root"=12] ("system directory type")
            n158 = Unbundle By Name(w354) -> ("Baseline.f0"=w332:dbl, "Baseline.df"=w340:dbl, "Baseline.magnitude"=w331:dbl[], "Audio.magnitude"=w330:dbl[], "Diff.magnitude"=w329:dbl[])
            n159 = Number To Fractional String(number=w332) -> (F-format string=w327:string)  [unwired: 3 in]
            n160 = Number To Fractional String(number=w330) -> (F-format string=w323:string[])  [unwired: 3 in]
            n161 = Number To Fractional String(number=w329) -> (F-format string=w322:string[])  [unwired: 3 in]
            n162 = Number To Fractional String(number=w340) -> (F-format string=w326:string)  [unwired: 3 in]
            n163 = Number To Fractional String(number=w331) -> (F-format string=w324:string[])  [unwired: 3 in]
            n164 = Format Date/Time String(time format string (%c)="Audio Data, %H%M%S_%m%d%Y.csv" ("prompt (Choose or enter file path)")) -> (date/time string=w342:string)  [unwired: 2 in]
            n165 = call <vilib>:"Get System Directory.vi"("system directory type"=w344) -> ("system directory"=w343:path)  [unwired: 10 in]
            n166 = Build Array(w326) -> (w325:string[])
            n167 = Build Array(w327) -> (w328:string[])
            n168 = Build Path(base path=w343, name or relative path=w342) -> (appended path=w341:path)
            n169 = Open/Create/Replace File(file path (use dialog)=w341, operation (0:open)=T10."replace or create") -> (refnum out=w350:refnum<file>, cancelled=w346:bool, error out=w353:errorcluster)  [unwired: 4 in]
            n170 = Build Array(w328, w325, w324, w323, w322) -> (w339:string[][])
            n171 = Transpose 2D Array(2D array=w339) -> (transposed array=w337:string[][])
            n172 = Build Array (concatenate)(string[] ["F0", "dF", "Baseline", "Audio", "Diff"], w337) -> (w336:string[][])
            n173 = Array To Spreadsheet String(delimiter (Tab)=",", array=w336, 3:"" ("format string")) -> (spreadsheet string=w333:string)
            n174 = Write to Text File(file (use dialog)=w350, text=w333, error in=w353) -> (refnum out=w351:refnum<file>, error out=w352:errorcluster)  [unwired: 1 in, 1 out]
            n175 = Close File(refnum=w351, error in=w352) -> (path=w349:path, error out=w348:errorcluster)
            n176 = case shown="False" w346 {
              tunnel: w349 -> [w357 _]
              tunnel: w348 -> [w356 _]
              frame False {
                n177 = call <vilib>:"File.Open File or Folder.vi"("Error In"=w356, "Path"=w357) -> ()  [unwired: 9 in, 1 out]
              }
              frame True {
              }
            }
          }
          frame "Return" {
            n178 = Variant To Data(type="", Variant=w359) -> (data=w364:string, error out=w363:errorcluster)  [unwired: 1 in]
            n179 = case shown="No Error" w363 {
              selector: w363 -> [_ w376]
              tunnel: w364 -> [w373 _]
              tunnel: [w371 w376] -> w360
              tunnel: w362 -> [w370 w375]
              tunnel: [w369 w375] -> w361
              tunnel: w358 -> [w367 _]
              frame No Error {
                n180 = Unbundle By Name(w370) -> ("FunctMgr"=w374:refnum<class "FunctMgr.lvclass">, "Local Error"=w368:errorcluster)
                n181 = call "FunctMgr.Pop and Return.vi"("error in (no error)"=w368, "Data"=w367, "Ret ID"=w373, "FunctMgr in"=w374) -> ("error out"=w371:errorcluster, "FunctMgr out"=w372:refnum<class "FunctMgr.lvclass">)  [unwired: 5 in, 1 out]
                n182 = Bundle By Name(cluster=w370, "FunctMgr"=w372) -> (w369:T15)
              }
              frame Error {
                # "Can't Return.  Invalid ID."
              }
            }
          }
          frame "Status" {
            n183 = Variant To Data(type="", Variant=w380) -> (data=w382:string, error out=w381:errorcluster)  [unwired: 1 in]
            n184 = case shown="No Error" w381 {
              selector: w381 -> [_ w388]
              tunnel: w379 -> [w387 _]
              tunnel: w378 -> [_ _]
              tunnel: w382 -> [w385 _]
              tunnel: [_ w388] -> w377
              frame No Error {
                # "Received from Child\nOnly write to status indicator (not event log)\nChild already recorded to event log."
                n185 = Unbundle By Name(w387) -> ("Log"=w386:refnum<class "Event Notification.lvclass">)
                n186 = call <vilib>:"Event Notification.Status Message.vi"("Log"=FALSE, "Message"=w385, "Event Notification in"=w386) -> ()  [unwired: 9 in]
              }
              frame Error {
              }
            }
          }
          frame Default {
            n187 = call <vilib>:"Module.Default Tasks.vi"("Sys"=w394, "error in"=w390, "Data2"=w391, "Data1"=w392, "Sub"=w393) -> ("error out"=w389:errorcluster)  [unwired: 5 in, 1 out]
          }
        }
      }
      frame "Function" {
        # "Return by default"
        n188 = case shown="\"Audio_GetResult\"" w404 {
          selector: w404 -> [w416 _ _ _ _ _]
          tunnel: w408 -> [w420 w425 w429 w436 w449 w477]
          tunnel: w407 -> [w421 w424 w428 w435 w448 w476]
          tunnel: [w420 w425 w429 w436 w449 w477] -> w406
          tunnel: [w421 w424 w428 w435 w448 w476] -> w405
          tunnel: w403 -> [_ _ _ w434 w447 _]
          tunnel: w402 -> [w417 w422 w427 _ _ _]
          tunnel: w401 -> [_ _ _ _ _ _]
          tunnel: w399 -> [w415 _ _ _ _ _]
          tunnel: [w414 _ _ _ _ _] -> w398
          tunnel: [variant _ _ _ _ w468] -> w397
          tunnel: [FALSE _ _ _ _ _] -> w396
          frame Default {
            n189 = call <vilib>:"SeqMgr.Error, Build Function Name Error Message.vi"("Data2"=w415, "Funct_Seq Name"=w416, "Local Q"=w417) -> ("error out"=w414:errorcluster)  [unwired: 8 in]
          }
          frame "Audio_ReadBaseline" {
            n190 = call <vilib>:"Q.Enqueue Task.vi"("Task Name"="Audio - Read Baseline", "Q In"=w422) -> ()  [unwired: 8 in, 2 out]
          }
          frame "Audio_ReadAudio" {
            n191 = call <vilib>:"Q.Enqueue Task.vi"("Task Name"="Audio - Read Audio", "Q In"=w427) -> ()  [unwired: 8 in, 2 out]
          }
          frame "Audio_SetDuration" {
            n192 = Variant To Data(type=string[] [], Variant=w434) -> (data=w431:string[], error out=w432:errorcluster)  [unwired: 1 in]
            n193 = case shown="No Error" w432 {
              tunnel: w431 -> [w441 _]
              tunnel: [w437 1.0 ("upper limit")] -> w430
              frame No Error {
                n194 = Index Array(array=w441) -> (element=w440:string)  [unwired: 1 in]
                n195 = Fract/Exp String To Number(string=w440) -> (number=w442:dbl)  [unwired: 3 in, 1 out]
                n196 = In Range and Coerce(upper limit=10.0, x=w442, lower limit=0.1 ("upper limit")) -> (coerced(x)=w437:dbl)  [unwired: 1 out]
              }
              frame Error {
              }
            }
            n197 = local write "Interval(s)"(w430) -> ()
          }
          frame "Audio_SetLimits" {
            n198 = Variant To Data(type=string[] [], Variant=w447) -> (data=w444:string[], error out=w445:errorcluster)  [unwired: 1 in]
            n199 = case shown="No Error" w445 {
              tunnel: w444 -> [w452 _]
              frame No Error {
                n200 = Array Size(array=w452) -> (size(s)=w456:i32)
                n201 = To Double Precision Float(number=w456) -> (double precision float=w455:dbl)
                n202 = Divide(x=w455, y=3.0) -> (x/y=w454:dbl)
                n203 = Fract/Exp String To Number(string=w452) -> (number=w451:dbl[])  [unwired: 3 in, 1 out]
                n204 = To Long Integer(number=w454) -> (32bit integer=w453:i32)
                n205 = for {
                  N: w453 -> [_]
                  tunnel: w451 -> [w464]
                  tunnel: [w458] -> w450 mode=indexing
                  i -> [w466]
                  n206 = Multiply(x=w466, y=3) -> (x*y=w463:i32)
                  n207 = Index Array(array=w464, index #1=w463) -> (element #1=w461:dbl, element #2=w460:dbl, element #3=w459:dbl)  [unwired: 2 in]
                  n208 = Bundle By Name(cluster=T11 {"FreqStart"=0.0, "FreqEnd"=1000.0, "Lim"=-45.0, "Result"=FALSE} ("Cluster"), "FreqStart"=w461, "FreqEnd"=w460, "Lim"=w459) -> (w458:T11)
                }
                n209 = local write "Limits"(w450) -> ()
              }
              frame Error {
                (unwired) 1.0 ("upper limit")
              }
            }
          }
          frame "Audio_GetResult" {
            n210 = local read "Limits"() -> (w474:T1)
            n211 = for {
              tunnel: w474 -> [w479] mode=indexing
              tunnel: [w478] -> w473 mode=indexing
              n212 = Unbundle By Name(w479) -> ("Result"=w478:bool)
            }
            n213 = And Array Elements(Boolean array=w473) -> (logical AND=w472:bool)
            n214 = Select(t="1", s=w472, f="0") -> (s? t:f=w469:string)
            n215 = Build Array("AudioResult", w469) -> (w467:string[])
            n216 = To Variant(anything=w467) -> (Variant=w468:variant)
          }
        }
        n217 = case shown="False" w396 {
          tunnel: [w412 w413] -> w400
          tunnel: w399 -> [w411 _]
          tunnel: w398 -> [w410 w413]
          tunnel: w397 -> [w409 _]
          frame False {
            n218 = call <vilib>:"Q.Return Function Data.vi"("error in"=w410, "Data2"=w411, "Ret Data"=w409) -> ("error out"=w412:errorcluster)  [unwired: 8 in]
          }
          frame True {
          }
        }
      }
      frame "App" {
        n219 = case shown="\"Set Logging Level\"" w487 {
          tunnel: w486 -> [_ _]
          tunnel: w485 -> [_ w499]
          tunnel: w484 -> [_ _]
          tunnel: w483 -> [w489 w496]
          tunnel: w482 -> [w488 w498]
          tunnel: [w489 w497] -> w481
          tunnel: [w488 w498] -> w480
          frame Default {
          }
          frame "Set Logging Level" {
            n220 = Variant To Data(type=Event_Log.Log_Level."Normal" ("Log Level"), Variant=w499) -> (data=w492:T2)  [unwired: 1 in, 1 out]
            n221 = local read "Logging Level"() -> (w491:T2)
            n222 = Unbundle By Name(w496) -> ("Log"=w494:refnum<class "Event Notification.lvclass">)
            n223 = Not Equal?(x=w492, y=w491) -> (x != y?=w490:bool)
            n224 = call <vilib>:"Event Notification.Set Logging Level.vi"("Log Level"=w492, "Event Notification in"=w494) -> ("Event Notification out"=w495:refnum<class "Event Notification.lvclass">)  [unwired: 9 in]
            n225 = case shown="True" w490 {
              tunnel: w492 -> [_ w500]
              frame False {
              }
              frame True {
                n226 = local write "Logging Level"(w500) -> ()
              }
            }
            n227 = Bundle By Name(cluster=w496, "Log"=w495) -> (w497:T7)
          }
        }
      }
      frame "Error", Default {
        n228 = case shown="\"Error\"" w508 {
          selector: w508 -> [_ w560]
          tunnel: [_ w561] -> w509
          tunnel: w507 -> [w518 _]
          tunnel: w506 -> [w516 _]
          tunnel: w505 -> [w517 _]
          tunnel: w504 -> [w515 _]
          tunnel: w502 -> [w512 w559]
          tunnel: w503 -> [w513 _]
          tunnel: [w511 w559] -> w501
          frame "Error" {
            n229 = case shown="\"Clear\"" w517 {
              tunnel: w518 -> [_ w557 _]
              tunnel: w516 -> [w553 _ _]
              tunnel: [w553 w555 _] -> w510
              tunnel: w515 -> [w552 w554 w558]
              tunnel: [w552 w554 w558] -> w514
              frame Default {
              }
              frame "Error" {
                n230 = Variant To Data(type=errorcluster {"status"=FALSE, "code"=0, "source"=""} ("error constant"), Variant=w557) -> (data=w555:errorcluster)  [unwired: 1 in, 1 out]
              }
              frame "Clear" {
              }
            }
            n231 = case shown="Error" w510 {
              selector: w510 -> [_ w531]
              tunnel: w514 -> [_ _]
              tunnel: w513 -> [w521 w534]
              tunnel: w512 -> [w524 w543]
              tunnel: [w523 w542] -> w511
              frame No Error {
                # "Clear Local Errors"
                n232 = Unbundle By Name(w524) -> ("Local Error"=w526:errorcluster)
                n233 = Unbundle By Name(w521) -> ("Log"=w520:refnum<class "Event Notification.lvclass">)
                n234 = case shown="Error" w526 {
                  tunnel: w520 -> [_ w530]
                  frame No Error {
                  }
                  frame Error {
                    n235 = call <vilib>:"Event Notification.Status Message.vi"("Display"=TRUE, "Level"=Event_Log.Log_Level."Normal", "Message"="Cleared Errors", "Event Notification in"=w530) -> ()  [unwired: 8 in]
                  }
                }
                n236 = control-ref of="Error Status"() -> (w522:refnum<vi>)
                n237 = invoke on="Error" class="Clust (strict)" method="Reinit To Default"() -> ()  [unwired: 3 in, 3 out]
                n238 = property on="Clear Error" class="Bool"("Visible"=FALSE) -> ()  [unwired: 2 in, 2 out]
                n239 = call <vilib>:"Status.Simple Text Status Indicator.vi"("Status TextBox"=w522) -> ()  [unwired: 10 in, 1 out]
                n240 = Bundle By Name(cluster=w524, "Local Error"=errorcluster {"status"=FALSE, "code"=0, "source"=""}) -> (w523:T15)
              }
              frame Error {
                # "Record Error"
                n241 = Unbundle By Name(w543) -> ("Local Error"=w541:errorcluster)
                n242 = Unbundle By Name(w534) -> ("Log"=w538:refnum<class "Event Notification.lvclass">)
                n243 = Unbundle By Name(w531) -> ("code"=w545:i32, "source"=w544:string)
                n244 = Unbundle By Name(w534) -> ("Cfg.Is Child?"=w533:bool, "Cfg.Parent Q"=w532:refnum<queue>)
                n245 = Format Into String(format string="ERROR!!! Code: %d, Desc: %s", w545, w544) -> (resulting string=w537:string)  [unwired: 2 in, 1 out]
                n246 = control-ref of="Error Status"() -> (w539:refnum<vi>)
                n247 = property on="Clear Error" class="Bool"("Visible"=TRUE) -> ()  [unwired: 2 in, 2 out]
                n248 = Merge Errors(w541, w531) -> (w540:errorcluster)
                n249 = call <vilib>:"Event Notification.Status Message with Error In.vi"("Type"=Event_Log.Notification_Type."Error", "Message"=w537, "Event Notification in"=w538) -> ()  [unwired: 9 in]
                n250 = call <vilib>:"Status.Simple Text Status Indicator.vi"("error in"=w531, "Status TextBox"=w539) -> ()  [unwired: 9 in, 1 out]
                n251 = case shown="True" w533 {
                  tunnel: w532 -> [_ w551]
                  tunnel: w531 -> [_ w550]
                  tunnel: [_ w547] -> _
                  frame False {
                  }
                  frame True {
                    w548 = "Error"
                    n252 = To Variant(anything=w550) -> (Variant=w549:variant)
                    n253 = call <vilib>:"Q.Enqueue Item.vi"("Data1"=w549, "Sub"=w548, "Cmd"=w548, "Q In"=w551) -> ("error out"=w547:errorcluster)  [unwired: 6 in, 1 out]
                  }
                }
                n254 = Bundle By Name(cluster=w543, "Local Error"=w540) -> (w542:T15)
                "Error" <- w531
              }
            }
          }
          frame Default {
            n255 = Concatenate Strings("Undefined State: \"", w560, "\".") -> (w562:string)
            n256 = Bundle By Name(cluster=errorcluster {"status"=TRUE, "code"=-5000, "source"=""} ("error constant"), "source"=w562) -> (w561:errorcluster)
          }
        }
      }
      frame "Exit" {
        # "This connection is made to not close\n the module until exit tasks are done."
        n257 = stacked-sequence {
          tunnel: w567 -> [w575 w577]
          tunnel: [errorcluster {"status"=FALSE, "code"=0, "source"=""} ("error constant") _] -> w566
          frame #0 {
            # "Close connection to instruments"
            n258 = Unbundle By Name(w575) -> ("Task ID"=w571:T13)
            n259 = call <vilib>:"Sound Input Stop.vi"("task ID"=w571) -> ("error out"=w573:errorcluster, "task ID out"=w572:T13)  [unwired: 9 in]
            n260 = call <vilib>:"Sound Input Clear.vi"("error in (no error)"=w573, "task ID"=w572) -> ("error out"=w574:errorcluster)  [unwired: 9 in]
            n261 = call <vilib>:"Clear Errors.vi"("error in (no error)"=w574) -> ()  [unwired: 5 in, 2 out]
          }
          frame #1 {
            # "Leave error not connected\nIgnore errors"
            # "Send Exit command to child modules"
            n262 = Unbundle By Name(w577) -> ("App.Child Modules"=w578:cluster{"VI Ref":refnum<vi>, "Name":string}[])
            n263 = for {
              tunnel: w578 -> [w581] mode=indexing
              tunnel: [w579] -> _ mode=indexing
              n264 = Unbundle By Name(w581) -> ("Name"=w580:string)
              n265 = call <vilib>:"Q.Enqueue Exit.vi"("Q Name"=w580) -> ("error out"=w579:errorcluster)  [unwired: 9 in, 1 out]
            }
          }
        }
        n266 = call <vilib>:"Module.Destructor.vi"("error in"=w566, "Sys"=w568) -> ("error out"=w570:errorcluster)  [unwired: 9 in]
      }
    }
  }
  n267 = while "Event Loop" {
    tunnel: w7 -> [w584]
    stop <- w585 stop-if-true
    n268 = Unbundle By Name(w584) -> ("Stop.Ref"=w583:refnum<event-registration>, "Main Q"=w582:refnum<queue>)
    n269 = event shown="[3] Menu Selection (User)" {
      selector: w583 -> [_ _ _ _ _ _ _ _ _ _ _]
      dyn-events: _ -> [_ _ _ _ _ _ _ _ _ _ _]
      timeout: _ -> [_ _ _ _ _ _ _ _ _ _ _]
      tunnel: [w592 _ _ w610 TRUE _ _ _ _ _ _] -> w585
      tunnel: w584 -> [w589 _ _ w608 _ _ _ _ _ _ _]
      tunnel: w582 -> [w594 w604 _ w609 _ w632 w633 w635 w637 w639 w644]
      event Panel Close? {
        n270 = event-data() -> ()  [unwired: 1 in, 4 out]
        n271 = Unbundle By Name(w589) -> ("Cfg.Parent Q"=w588:refnum<queue>)
        n272 = Unbundle By Name(w589) -> ("Cfg.Is Child?"=w590:bool)
        n273 = Not A Number/Path/Refnum?(number/path/refnum=w588) -> (NaN/Path/Refnum?=w587:bool)
        n274 = Not(x=w587) -> (.not. x?=w586:bool)
        n275 = And(x=w590, y=w586) -> (x .and. y?=w591:bool)
        n276 = case shown="True" w591 {
          tunnel: w594 -> [w597 w600]
          tunnel: [TRUE TRUE] -> w593
          tunnel: [TRUE FALSE] -> w592
          tunnel: [_ w598] -> _
          frame False {
            # "Parent - Exit"
            n277 = call <vilib>:"Q.Enqueue Exit.vi"("Q In"=w597) -> ()  [unwired: 9 in, 2 out]
          }
          frame True {
            # "Child - Hide Panel and if was \nin a subpanel, return to subpanel."
            n278 = call <vilib>:"Module.Window, Q Task.vi"("Action"=Window.Task,_Action."Return to SubPanel()", "Q In"=w600) -> ("error out"=w598:errorcluster)  [unwired: 8 in, 1 out]
          }
        }
        n279 = event-data("Discard?"=w593) -> ()  [unwired: 1 in, 1 out]
      }
      event Panel Resize {
        n280 = event-data() -> ()  [unwired: 1 in, 8 out]
        n281 = call <vilib>:"Module.Window, Q Task.vi"("Action"=Window.Task,_Action."Resize()", "Q In"=w604) -> ()  [unwired: 8 in, 2 out]
      }
      event "Leave Maint": Value Change {
        n282 = event-data() -> ()  [unwired: 1 in, 6 out]
        n283 = local write "Main Tab"(0) -> ()
      }
      event Menu Selection (User) {
        n284 = event-data() -> ("MenuRef"=w606:refnum<k9>, "ItemTag"=w607:string)  [unwired: 1 in, 5 out]
        n285 = case shown="\"Go to Maint Tab\"" w607 {
          selector: w607 -> [w612 _ _ _ _ w622 _ _]
          tunnel: [_ TRUE _ _ _ _ _ _] -> w610
          tunnel: w609 -> [_ w615 _ w618 _ w626 w628 w630]
          tunnel: [_ _ w617 _ _ _ _ _] -> _
          tunnel: w608 -> [w611 _ _ _ w620 _ _ _]
          tunnel: w606 -> [_ _ _ _ _ w623 _ _]
          frame Default {
            # "Check if a help document was selected.\nIf so, open the document"
            n286 = Unbundle By Name(w611) -> ("Docs.Tags"=w614:string[], "Docs.Paths"=w613:path[])
            n287 = call <vilib>:"Menu.Help, Open User Manual Items.vi"("Menu Tag Selection"=w612, "Paths"=w613, "Tags"=w614) -> ()  [unwired: 8 in, 1 out]
          }
          frame "Exit" {
            n288 = call <vilib>:"Q.Enqueue Exit.vi"("Q In"=w615) -> ()  [unwired: 9 in, 2 out]
          }
          frame "Event Log" {
            n289 = call <vilib>:"Event Log.Show.vi"() -> ("error out"=w617:errorcluster)  [unwired: 11 in]
          }
          frame "Reset" {
            n290 = call <vilib>:"Q.Enqueue Reset.vi"("Q In"=w618) -> ()  [unwired: 9 in, 2 out]
          }
          frame "Help.About" {
            n291 = Unbundle By Name(w620) -> ("SW Rev"=w619:T6)
            n292 = call <vilib>:"Help.About.vi"("SW Version"=w619) -> ()  [unwired: 11 in]
          }
          frame "Simulate OFF", "Simulate ON" {
            n293 = call <vilib>:"Menu.Simulate, Set Menu State.vi"("Menu Tag"=w622, "Menu Ref"=w623) -> ("Sim ON"=w621:bool)  [unwired: 8 in, 1 out]
            n294 = To Variant(anything=w621) -> (Variant=w625:variant)
            n295 = call <vilib>:"Q.Enqueue Task.vi"("Data1"=w625, "Task Name"="Simulate", "Q In"=w626) -> ()  [unwired: 7 in, 2 out]
          }
          frame "Show Block Diagram" {
            n296 = call <vilib>:"Module.Window, Q Task.vi"("Action"=Window.Task,_Action."Open Block Diagram()", "Q In"=w628) -> ()  [unwired: 8 in, 2 out]
          }
          frame "Go to Maint Tab" {
            n297 = call <vilib>:"Module.Window, Q Task.vi"("Action"=Window.Task,_Action."Go To Maint Tab()", "Q In"=w630) -> ()  [unwired: 8 in, 2 out]
          }
        }
      }
      event User Event {
        n298 = event-data() -> ()  [unwired: 1 in, 5 out]
      }
      event "Clear Error": Value Change {
        n299 = event-data() -> ()  [unwired: 1 in, 6 out]
        n300 = call "Error.Clear.vi"("Q In"=w632) -> ()  [unwired: 9 in, 2 out]
      }
      event "Read Audio": Value Change {
        n301 = event-data() -> ()  [unwired: 1 in, 6 out]
        n302 = call <vilib>:"Q.Enqueue Task.vi"("Task Name"="Audio - Read Audio" ("Name"), "Q In"=w633) -> ()  [unwired: 8 in, 2 out]
      }
      event "Read Baseline": Value Change {
        n303 = event-data() -> ()  [unwired: 1 in, 6 out]
        n304 = call <vilib>:"Q.Enqueue Task.vi"("Task Name"="Audio - Read Baseline" ("Name"), "Q In"=w635) -> ()  [unwired: 8 in, 2 out]
      }
      event "Toggle Sim": Value Change {
        n305 = event-data() -> ()  [unwired: 1 in, 6 out]
        n306 = call <vilib>:"Q.Enqueue Task.vi"("Task Name"="Simulate - Toggle" ("Name"), "Q In"=w637) -> ()  [unwired: 8 in, 2 out]
      }
      event "Save Data to File": Value Change {
        n307 = event-data() -> ()  [unwired: 1 in, 6 out]
        n308 = call <vilib>:"Q.Enqueue Task.vi"("Task Name"="Save Data to File", "Q In"=w639) -> ()  [unwired: 8 in, 2 out]
      }
      event Value Change {
        n309 = event-data() -> ()  [unwired: 1 in, 6 out]
        n310 = To Variant(anything="Logging Level") -> (Variant=w642:variant)
        n311 = call <vilib>:"Q.Enqueue Task.vi"("Data1"=w642, "Task Name"="Set Logging Level", "Q In"=w644) -> ()  [unwired: 7 in, 2 out]
      }
    }
  }
